vi "Publish Error Image.vi"(8 "error in (no error)":errorcluster, 11 "Camera Actor in":refnum<class "Camera Actor.lvclass">) -> (0 "error out":errorcluster, 3 "Camera Actor out":refnum<class "Camera Actor.lvclass">)   [LabVIEW 2020, in "Camera Actor.lvlib" / "Camera Actor.lvclass"]
uses:
  Camera Actor.lvclass
  C:/Program Files (x86)/National Instruments/LabVIEW 2020/vi.lib/ActorFramework/Actor/Actor.lvclass
  <vilib>/Utility/error.llb/DialogType.ctl
  Camera Actor.lvclass/Camera Actor.ctl
  <vilib>/ActorFramework/Message Enqueuer/Message Priority.ctl
  <vilib>/ActorFramework/Actor/Actor.lvclass/Actor.ctl
  <vilib>/ActorFramework/Message Enqueuer/Message Enqueuer.lvclass/Message Enqueuer.ctl
  <vilib>/ActorFramework/Report Error Msg/Report Error Msg.lvclass/Report Error Msg.ctl
  <vilib>/ActorFramework/Message Enqueuer/Init from Existing Queue.vi
  <vilib>/ActorFramework/Message Enqueuer/Enqueue.vi
  <vilib>/ActorFramework/Report Error Msg/Report Error Msg.lvclass
  C:/Program Files (x86)/National Instruments/LabVIEW 2020/vi.lib/ActorFramework/Message/Message.lvclass
  <vilib>/ActorFramework/Message Priority Queue/Priority Enqueue.vi
  <vilib>/ActorFramework/Message Enqueuer/Message Enqueuer.lvclass
  <vilib>/ActorFramework/Actor/Actor.lvclass
panel:
  in  "Comment":string
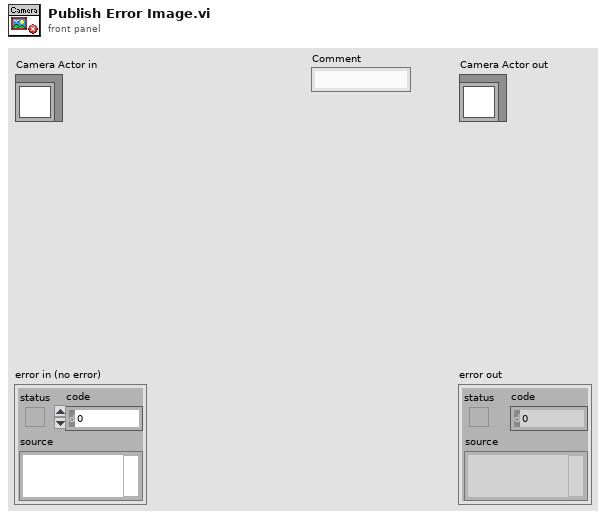
[diagram p1: front panel]
types:
  T1 = cluster{"Desired Font (Application)":enum16{"User-specified Font", "Application Font", "System Font", "Dialog Font"}, "[User-specified Font]":cluster{"Font Name":string, "Size":i16, "Strikeout?":bool, "Italic?":bool, "Underline?":bool, "Outline?":bool, "Shadow?":bool, "Bold?":bool, "Rotation Angle":dbl}, "Horizontal Alignment":i16, "Vertical Alignment":i16}
  T2 = typedef "Actor Framework.lvlib/Message Enqueuer.lvclass/Message Priority.ctl" = enum16{"Low", "Normal", "High"}
  T3 = typedef "DialogType.ctl" = u16
  T4 = typedef "IMAQ Image.ctl" = refnum<image>
  T5 = typedef "Camera Actor.lvlib/Camera Actor.lvclass/Operation Mode.ctl" = enum16{"Run", "Stop", "Exit", "Error", "Restart"}
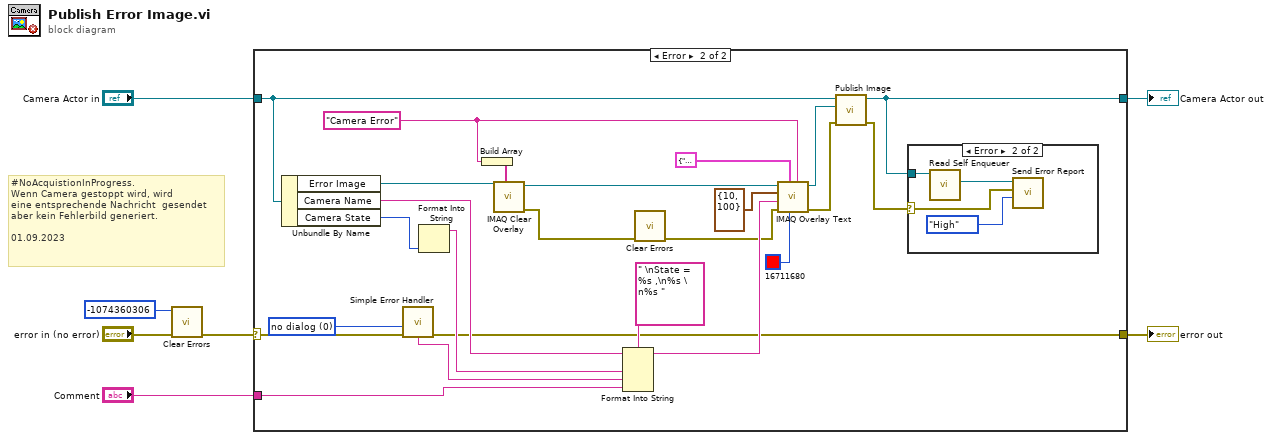
[diagram p0: block diagram]
diagram:
  # "#NoAcquistionInProgress.\nWenn Camera gestoppt wird, wird\neine entsprechende Nachricht  gesendet\naber kein Fehlerbild generiert.\n\n01.09.2023"
  n1 = call <vilib>:"Clear Errors.vi"("error in (no error)"="error in (no error)", "specific error code to clear (0: all)"=-1074360306 ("Code")) -> ("error out"=w2:errorcluster)  [unwired: 4 in, 1 out]
  n2 = case shown="Error" w2 {
    selector: w2 -> [w9 w11]
    tunnel: [w9 w10] -> w6
    tunnel: [w8 w18] -> w4
    tunnel: "Camera Actor in" -> [w8 w22]
    tunnel: "Comment" -> [_ w24]
    frame No Error {
    }
    frame Error {
      w13 = T3 0 items=["no dialog", "OK message", "continue or stop message", "OK message + warnings", "continue/stop + warnings"] ("type of dialog (OK msg:1)")
      w28 = "Camera Error" ("Group")
      n3 = Unbundle By Name(w22) -> ("Error Image"=w15:T4, "Camera Name"=w32:string, "Camera State"=w25:T5)
      n4 = call <vilib>:"Simple Error Handler.vi"("type of dialog (OK msg:1)"=w13, "error in (no error)"=w11) -> ("error out"=w10:errorcluster, "message"=w12:string)  [unwired: 3 in, 3 out]
      n5 = Format Into String(w25) -> (resulting string=w31:string)  [unwired: 3 in, 1 out]
      n6 = Build Array(w28) -> (w27:string[])
      n7 = call "IMAQ Clear Overlay"("Groups"=w27, "Image"=w15) -> ("error out"=w23:errorcluster, "Image Out"=w29:T4)  [unwired: 8 in]
      n8 = Format Into String(format string=" \nState = %s ,\n%s \n%s ", initial string=w32, w31, w12, w24) -> (resulting string=w33:string)  [unwired: 1 in, 1 out]
      n9 = call <vilib>:"Clear Errors.vi"("error in (no error)"=w23) -> ("error out"=w14:errorcluster)  [unwired: 5 in, 1 out]
      n10 = call "IMAQ Overlay Text"("Group"=w28, "Text Color (black)"=u32 16711680, "Font, Size & Style"=T1 {"Desired Font (Application)"=enum."User-specified Font", "[User-specified Font]"={"Font Name"="", "Size"=22, "Strikeout?"=FALSE, "Italic?"=FALSE, "Underline?"=FALSE, "Outline?"=FALSE, "Shadow?"=FALSE, "Bold?"=TRUE, "Rotation Angle"=0.0}, "Horizontal Alignment"=0, "Vertical Alignment"=0}, "error in (no error)"=w14, "String"=w33, "Origin"=cluster{"X":i32, "Y":i32} {"X"=10, "Y"=100}, "Image"=w29) -> ("error out"=w20:errorcluster, "Image Out"=w21:T4)  [unwired: 3 in]
      n11 = call-dynamic "Publish Image.vi"("error in (no error)"=w20, "Image"=w21, "Camera in"=w22) -> ("error out"=w19:errorcluster, "Camera out"=w18:refnum<class "Camera Actor.lvclass">)  [unwired: 7 in]
      n12 = case shown="Error" w19 {
        selector: w19 -> [_ w35]
        tunnel: w18 -> [_ w37]
        frame No Error {
        }
        frame Error {
          n13 = call <vilib>:"Read Self Enqueuer.vi"("Actor"=w37) -> ("Self Enqueuer"=w36:refnum<class "Message Enqueuer.lvclass">)  [unwired: 10 in]
          n14 = call <vilib>:"Send Error Report.vi"("Message Priority (Normal)"=Message_Priority."High", "Error From Sender"=w35, "Message Enqueuer"=w36) -> ()  [unwired: 8 in, 1 out]
        }
      }
    }
  }
  "error out" <- w6
  "Camera Actor out" <- w4
